vi "XY Plot Commands W2D.vi"(0 "wavenames":string[](array[string])=["'IV0_summ.itx.0003'[0][0]", "'IV0_summ.itx.0003'[0][1]", "'IV0_summ.itx.0003'[0][2]", "'IV0_summ.itx.0003'[0][3]", "'IV0_summ.itx.0003'[0][4]", "'IV0_summ.itx.0003'[0][5]", "'IV0_summ.itx.0003'[0][6]", "'IV0_summ.itx.0003'[0][7]", "'IV0_summ.itx.0003'[0][8]", "'IV0_summ.itx.0003'[0][9]", "'IV0_summ.itx.0003'[0][10]", "'IV0_summ.itx.0003'[0][11]", "'IV0_summ.itx.0003'[0][12]", "'IV0_summ.itx.0003'[0][13]", "'IV0_summ.itx.0003'[0][14]", "'IV0_summ.itx.0003'[0][15]", "'IV0_summ.itx.0003'[0][16]", "'IV0_summ.itx.0003'[0][17]", "'IV0_summ.itx.0003'[0][18]", "'IV0_summ.itx.0003'[0][19]", "'IV0_summ.itx.0003'[0][20]"], 1 "X label":string="energy (eV)", 2 "Y label":string="amplitude (arb)", 3 "input string":string="Display #wave# vs '#waveX#'\nAppendToGraph #wave# vs '#waveX#'\nLabel bottom \"#labelX#\"\nLabel left \"#labelY#\"\nModifyGraph rgb(#wave#)=(#r#,#g#,#b#)\nLegend/C/N=text0\nModifyGraph mirror=1", 4 "X wave":string="x_") -> (5 "result string":string="Display 'IV0_summ.itx.0003'[0][0] vs 'x_'\nAppendToGraph 'IV0_summ.itx.0003'[0][1] vs 'x_'\nAppendToGraph 'IV0_summ.itx.0003'[0][2] vs 'x_'\nAppendToGraph 'IV0_summ.itx.0003'[0][3] vs 'x_'\nAppendToGraph 'IV0_summ.itx.0003'[0][4] vs 'x_'\nAppendToGraph 'IV0_summ.itx.0003'[0][5] vs 'x_'\nAppendToGraph 'IV0_summ.itx.0003'[0][6] vs 'x_'\nAppendToGraph 'IV0_summ.itx.0003'[0][7] vs 'x_'\nAppendToGraph 'IV0_summ.itx.0003'[0][8] vs 'x_'\nAppendToGraph 'IV0_summ.itx.0003'[0][9] vs 'x_'\nAppendToGraph 'IV0_summ.itx.0003'[0][10] vs 'x_'\nAppendToGraph 'IV0_summ.itx.0003'[0][11] vs 'x_'\nAppendToGraph 'IV0_summ.itx.0003'[0][12] vs 'x_'\nAppendToGraph 'IV0_summ.itx.0003'[0][13] vs 'x_'\nAppendToGraph 'IV0_summ.itx.0003'[0][14] vs 'x_'\nAppendToGraph 'IV0_summ.itx.0003'[0][15] vs 'x_'\nAppendToGraph 'IV0_summ.itx.0003'[0][16] vs 'x_'\nAppendToGraph 'IV0_summ.itx.0003'[0][17] vs 'x_'\nAppendToGraph 'IV0_summ.itx.0003'[0][18] vs 'x_'\nAppendToGraph 'IV0_summ.itx.0003'[0][19] vs 'x_'\nAppendToGraph 'IV0_summ.itx.0003'[0][20] vs 'x_'\nLabel bottom \"energy (eV)\"\nLabel left \"amplitude (arb)\"\nModifyGraph rgb('IV0_summ.itx.0003'[0][0])=(65280,0,0)\nModifyGraph rgb('IV0_summ.itx.0003'[0][1])=(65280,16896,0)\nModifyGraph rgb('IV0_summ.itx.0003'[0][2])=(65280,33792,0)\nModifyGraph rgb('IV0_summ.itx.0003'[0][3])=(65280,50688,0)\nModifyGraph rgb('IV0_summ.itx.0003'[0][4])=(63488,65280,0)\nModifyGraph rgb('IV0_summ.itx.0003'[0][5])=(46592,65280,0)\nModifyGraph rgb('IV0_summ.itx.0003'[0][6])=(29696,65280,0)\nModifyGraph rgb('IV0_summ.itx.0003'[0][7])=(12800,65280,0)\nModifyGraph rgb('IV0_summ.itx.0003'[0][8])=(0,65280,4096)\nModifyGraph rgb('IV0_summ.itx.0003'[0][9])=(0,65280,20992)\nModifyGraph rgb('IV0_summ.itx.0003'[0][10])=(0,65280,37888)\nModifyGraph rgb('IV0_summ.itx.0003'[0][11])=(0,65280,53248)\nModifyGraph rgb('IV0_summ.itx.0003'[0][12])=(0,60928,65280)\nModifyGraph rgb('IV0_summ.itx.0003'[0][13])=(0,44032,65280)\nModifyGraph rgb('IV0_summ.itx.0003'[0][14])=(0,27136,65280)\nModifyGraph rgb('IV0_summ.itx.0003'[0][15])=(0,10240,65280)\nModifyGraph rgb('IV0_summ.itx.0003'[0][16])=(6656,0,65280)\nModifyGraph rgb('IV0_summ.itx.0003'[0][17])=(23552,0,65280)\nModifyGraph rgb('IV0_summ.itx.0003'[0][18])=(40448,0,65280)\nModifyGraph rgb('IV0_summ.itx.0003'[0][19])=(57344,0,65280)\nModifyGraph rgb('IV0_summ.itx.0003'[0][20])=(65280,0,56832)\nLegend/C/N=text0")   [LabVIEW 2019, in "Data.ITX.lvclass"]
uses:
  Data.ITX.lvclass
  Graph Utilities/graph_utilities.lvclass
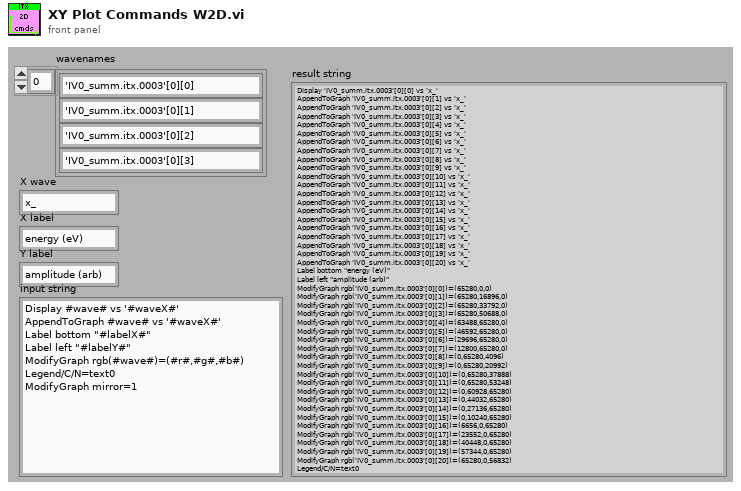
[diagram p1: front panel]
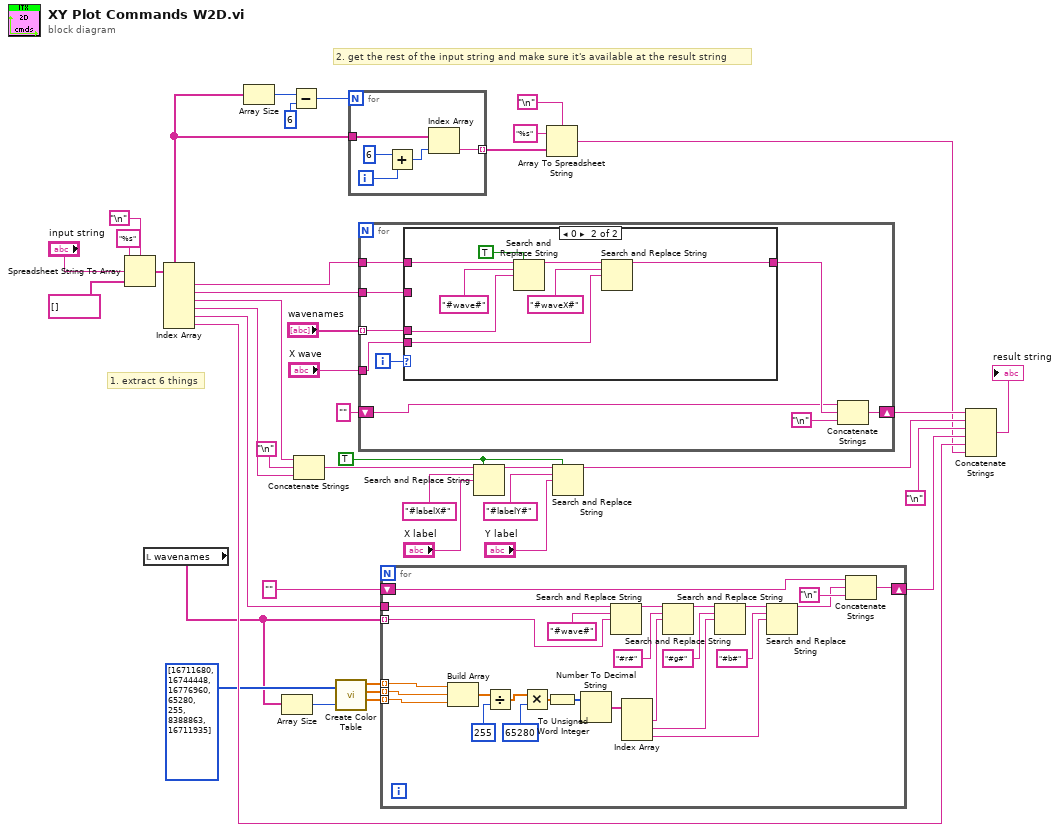
[diagram p0: block diagram]
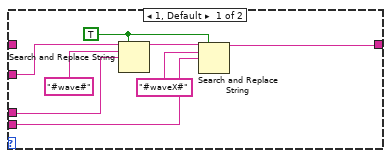
[diagram p2: hidden frame]
diagram:
  w24 = TRUE ("replace all? (F)")
  # "2. get the rest of the input string and make sure it's available at the result string"
  # "1. extract 6 things"
  n1 = Spreadsheet String To Array(delimiter (Tab)="\n", format string="%s", spreadsheet string="input string", array type (2D Dbl)=string[] []) -> (array=w8:string[])
  n2 = local read "wavenames"() -> (w1:string[])
  n3 = Index Array(array=w8) -> (element #1=w32:string, element #2=w31:string, element #3=w15:string, element #4=w16:string, element #5=w17:string, element #6=w18:string)  [unwired: 6 in]
  n4 = Array Size(array=w8) -> (size(s)=w14:i32)
  n5 = Array Size(array=w1) -> (size(s)=w6:i32)
  n6 = Subtract(x=w14, y=6 ("x")) -> (x-y=w12:i32)
  n7 = Concatenate Strings(w15, "\n", w16) -> (w29:string)
  n8 = call "Create Color Table.vi"("Colors []"=u32[] [16711680, 16744448, 16776960, 65280, 255, 8388863, 16711935], "Size (256)"=w6) -> ("R []"=w5:dbl[], "G []"=w4:dbl[], "B []"=w3:dbl[])  [unwired: 1 out]
  n9 = for {
    N: w12 -> [_]
    tunnel: w8 -> [w43]
    tunnel: [w42] -> w11 mode=indexing
    i -> [w45]
    n10 = Add(x=6, y=w45) -> (x+y=w46:i32)
    n11 = Index Array(array=w43, index=w46) -> (element=w42:string)
  }
  n12 = for {
    tunnel: "wavenames" -> [w53] mode=indexing
    tunnel: w32 -> [w55]
    tunnel: w31 -> [w54]
    shift-right: [w51] -> w36
    shift-left: "" -> [w48]
    tunnel: "X wave" -> [w47]
    i -> [w52]
    n13 = case shown="0" w52 {
      tunnel: w55 -> [_ w69]
      tunnel: w54 -> [w61 _]
      tunnel: w53 -> [w62 w70]
      tunnel: [w57 w66] -> w50
      tunnel: w47 -> [w58 w64]
      frame 1, Default {
        w56 = TRUE ("replace all? (F)")
        n14 = Search and Replace String(replace all?=w56, input string=w61, search string="#wave#", replace string=w62) -> (result string=w60:string)  [unwired: 1 in, 6 out]
        n15 = Search and Replace String(replace all?=w56, input string=w60, search string="#waveX#", replace string=w58) -> (result string=w57:string)  [unwired: 1 in, 6 out]
      }
      frame 0 {
        n16 = Search and Replace String(replace all?=TRUE ("replace all? (F)"), input string=w69, search string="#wave#", replace string=w70) -> (result string=w67:string)  [unwired: 1 in, 6 out]
        n17 = Search and Replace String(input string=w67, search string="#waveX#", replace string=w64) -> (result string=w66:string)  [unwired: 1 in, 7 out]
      }
    }
    n18 = Concatenate Strings(w48, w50, "\n") -> (w51:string)
  }
  n19 = for {
    tunnel: w17 -> [w90]
    tunnel: w1 -> [w75] mode=indexing
    shift-right: [w86] -> w22
    shift-left: "" -> [w85]
    tunnel: w5 -> [w74] mode=indexing
    tunnel: w4 -> [w73] mode=indexing
    tunnel: w3 -> [w72] mode=indexing
    n20 = Build Array(w74, w73, w72) -> (w97:dbl[])
    n21 = Divide(x=w97, y=255) -> (x/y=w93:dbl[])
    n22 = Multiply(x=w93, y=65280) -> (x*y=w94:dbl[])
    n23 = To Unsigned Word Integer(number=w94) -> (unsigned 16bit integer=w92:u16[])
    n24 = Number To Decimal String(number=w92) -> (decimal integer string=w79:string[])  [unwired: 1 out]
    n25 = Search and Replace String(input string=w90, search string="#wave#", replace string=w75) -> (result string=w91:string)  [unwired: 1 in, 7 out]
    n26 = Index Array(array=w79) -> (element #1=w78:string, element #2=w77:string, element #3=w76:string)  [unwired: 3 in]
    n27 = Search and Replace String(input string=w91, search string="#r#", replace string=w78) -> (result string=w89:string)  [unwired: 1 in, 7 out]
    n28 = Search and Replace String(input string=w89, search string="#g#", replace string=w77) -> (result string=w88:string)  [unwired: 1 in, 7 out]
    n29 = Search and Replace String(input string=w88, search string="#b#", replace string=w76) -> (result string=w83:string)  [unwired: 1 in, 7 out]
    n30 = Concatenate Strings(w85, w83, "\n") -> (w86:string)
  }
  n31 = Search and Replace String(replace all?=w24, input string=w29, search string="#labelX#", replace string="X label") -> (result string=w27:string)  [unwired: 1 in, 6 out]
  n32 = Array To Spreadsheet String(delimiter (Tab)="\n", array=w11, 3:"%s" ("format string")) -> (spreadsheet string=w7:string)
  n33 = Search and Replace String(replace all?=w24, input string=w27, search string="#labelY#", replace string="Y label") -> (result string=w20:string)  [unwired: 1 in, 6 out]
  n34 = Concatenate Strings(w36, w20, "\n", w22, w18, w7) -> (→"result string":string)
